vi "move category to end.vi"(6 "Category":string, 7 "Sort by":T1, 9 "subnodes category in":string[](array[string]), 10 "subnodes class in":string[](array[string]), 11 "subnodes menu name in":string[](array[string])) -> (1 "subnodes category out":string[](array[string]), 2 "subnodes class out":string[](array[string]), 3 "subnodes menu name out":string[](array[string]))   [LabVIEW 2013, in "PL Framework Configuration Tool.lvlib" / "Engine Parent Editor Node.lvclass"]
uses:
  Engine Parent Editor Node.lvclass
  subnodes sort by.ctl
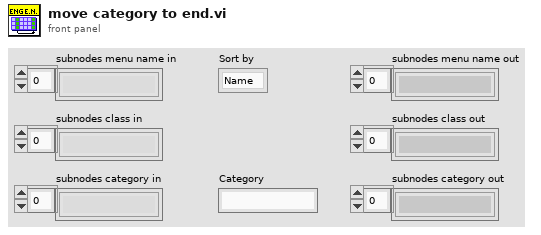
[diagram p1: front panel]
types:
  T1 = typedef "PL Framework Configuration Tool.lvlib/Engine Parent Editor Node.lvclass/subnodes sort by.ctl" = enum16{"Name", "Class", "Category"}
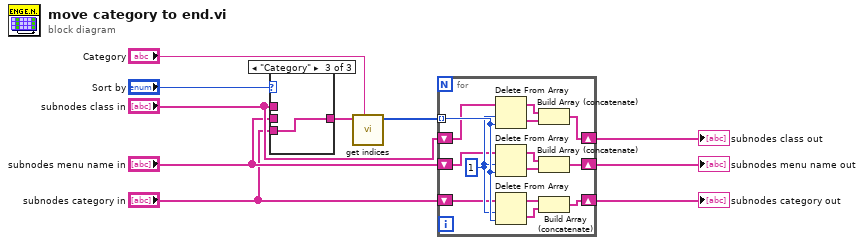
[diagram p0: block diagram]
diagram:
  n1 = case shown="\"Category\"" "Sort by" {
    tunnel: "subnodes class in" -> [_ w12 _]
    tunnel: [w11 w12 w13] -> w4
    tunnel: "subnodes menu name in" -> [w11 _ _]
    tunnel: "subnodes category in" -> [_ _ w13]
    frame "Name", Default {
    }
    frame "Class" {
    }
    frame "Category" {
    }
  }
  n2 = call "get indices.vi"("Category"="Category", "array in"=w4) -> ("Indices"=w1:i32[])  [unwired: 9 in]
  n3 = for {
    tunnel: w1 -> [w27] mode=indexing
    shift-right: [w16] -> w8
    shift-left: "subnodes menu name in" -> [w25]
    shift-right: [w15] -> w9
    shift-left: "subnodes class in" -> [w24]
    shift-right: [w14] -> w10
    shift-left: "subnodes category in" -> [w23]
    w26 = 1 ("length")
    n4 = Delete From Array(array=w24, length=w26, index=w27) -> (deleted portion=w19:string[], array with subset deleted=w20:string[])
    n5 = Delete From Array(array=w25, length=w26, index=w27) -> (deleted portion=w21:string[], array with subset deleted=w22:string[])
    n6 = Delete From Array(array=w23, length=w26, index=w27) -> (deleted portion=w17:string[], array with subset deleted=w18:string[])
    n7 = Build Array (concatenate)(w20, w19) -> (w15:string[])
    n8 = Build Array (concatenate)(w22, w21) -> (w16:string[])
    n9 = Build Array (concatenate)(w18, w17) -> (w14:string[])
  }
  "subnodes category out" <- w10
  "subnodes class out" <- w9
  "subnodes menu name out" <- w8
